vi "To XML - Returns XML Entities.vi"() -> ()   [LabVIEW 2017, in "Cobertura.Tests.lvlib" / "Package.lvlib"]
uses:
  Package.lvlib
  <vilib>/xml/Close Reference(Node).vi
  Cobertura/Package/Package.lvclass
  <vilib>/xml/NI_XML.lvlib
  <resource>/objmgr/DOMUserDefRef.rc
  <vilib>/PNR/Transparent Assertions/Transparent Assertions/Transparent Assertions.lvlib
panel:
  out "error out":errorcluster
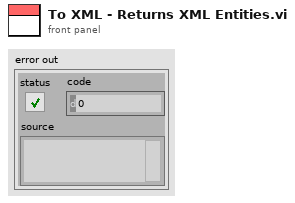
[diagram p1: front panel]
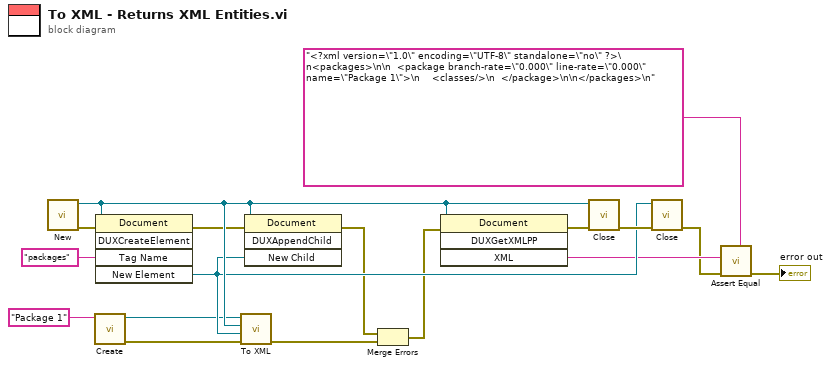
[diagram p0: block diagram]
diagram:
  n1 = call <vilib>:"New.vi"() -> ("error out"=w12:errorcluster, "DOM document out"=w14:refnum<k20>)  [unwired: 8 in]
  n2 = call "Create.vi"("Name"="Package 1") -> ("error out"=w17:errorcluster, "Package"=w1:refnum<class "Package.lvclass">)  [unwired: 9 in]
  n3 = invoke class="Document" method="DUXCreateElement"(reference=w14, error in=w12, "Tag Name"="packages") -> (error out=w13:errorcluster, "New Element"=w10:refnum<k20>)  [unwired: 2 in, 3 out]
  n4 = call-dynamic "To XML.vi"("error in (no error)"=w17, "Parent"=w10, "Document"=w14, "Package in"=w1) -> ("error out"=w4:errorcluster)  [unwired: 7 in]
  n5 = invoke class="Document" method="DUXAppendChild"(reference=w14, error in=w13, "New Child"=w10) -> (error out=w6:errorcluster)  [unwired: 1 in, 3 out]
  n6 = Merge Errors(w6, w4) -> (w5:errorcluster)
  n7 = invoke class="Document" method="DUXGetXMLPP"(reference=w14, error in=w5) -> (error out=w15:errorcluster, "XML"=w9:string)  [unwired: 2 in, 2 out]
  n8 = call-poly <vilib>:"Close.vi"("error in (no error)"=w15, "node"=w14) -> ("error out"=w11:errorcluster)  [unwired: 7 in]
  n9 = call-poly <vilib>:"Close.vi"("error in (no error)"=w11, "node"=w10) -> ("error out"=w3:errorcluster)  [unwired: 7 in]
  n10 = call <vilib>:"Assert Equal.vi"("Expected"="<?xml version=\"1.0\" encoding=\"UTF-8\" standalone=\"no\" ?>\n<packages>\n\n  <package branch-rate=\"0.000\" line-rate=\"0.000\" name=\"Package 1\">\n    <classes/>\n  </package>\n\n</packages>\n", "error in (no error)"=w3, "Actual"=w9) -> ("error out"=→"error out":errorcluster)  [unwired: 8 in]
